vi "Configure dB.vi"(0 "VISA resource name":refnum<visa-resource-name>, 5 "error in (no error)":errorcluster, 6 "State":bool, 9 "dB Reference":dbl min=0.0 max=200.0) -> (14 "VISA resource name out":refnum<visa-resource-name>, 19 "error out":errorcluster)   [LabVIEW 2020, in "Keithley 2100 Series.lvlib"]
doc: "Definition:\nThe dB feature takes a DC or AC voltage measurement and displays it in decibel unit in correspondence to a relative reference value. The calculation of dB is listed below:\n dB =20 log( Vin/Vref )\n or\n dB = (Input signal in dBm) – (relative value in dBm)\n\nNOTE: The in V is the input signal and the ref V is the relative reference.\n\nThe dB measurement is applied to DC and AC voltage only. The relative value is adjustable and is stored in a volatile memory. The range for the relative value is between 0 dBm and 200 dBm.\n\nHow to set the relative value:\nUser can either manually select a number for the relative reference or let the multimeter take the first reading (0 dB).\n\nRemote Interface Operation\n\nUse the following commands from your PC terminal to make the dB measurement:\n\nCALCulate:FUNCtion DB\nCALCulate:STATe {OFF|ON}\nCALCulate:STATe?\nCALCulate:DB:REFerence {<value>|MINimum|MAXimum}"
uses:
  Keithley 2100 Series.lvlib
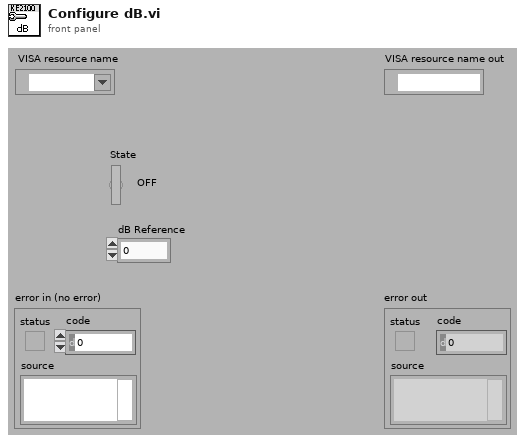
[diagram p1: front panel]
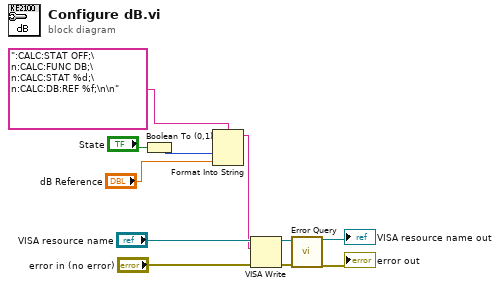
[diagram p0: block diagram]
diagram:
  n1 = Boolean To (0,1)(Boolean="State") -> (0, 1=w4:i16)
  n2 = Format Into String(format string=":CALC:STAT OFF;\n:CALC:FUNC DB;\n:CALC:STAT %d;\n:CALC:DB:REF %f;\n\n", w4, "dB Reference") -> (resulting string=w5:string)  [unwired: 2 in, 1 out]
  n3 = VISA Write(VISA resource name="VISA resource name", write buffer=w5, error in (no error)="error in (no error)") -> (VISA resource name out=w10:refnum<visa-resource-name>, error out=w11:errorcluster)  [unwired: 1 out]
  n4 = call "Error Query.vi"("VISA resource name"=w10, "error in (no error)"=w11) -> ("VISA resource name out"=→"VISA resource name out":refnum<visa-resource-name>, "error out"=→"error out":errorcluster)  [unwired: 14 in, 2 out]
